vi "_File Server.vi"(4 "Sample Info":string[](array[string]), 5 "AcqMethod":T1[](array[typedef]) {"ScanType" format="%#.6g"; "Mass Range"."Res" items=["High/High", "Medium/Medium", "Low/Low", "High/Medium", "High/Low", "Medium/High", "Medium/Low", "Low/High", "Low/Medium"]}, 7 "file path":path, 8 "error in (no error)":errorcluster, 9 "Scan#":i32=1, 10 "Spectrum":u32[](array[numeric]), 11 "File Command":T6) -> (0 "error out":errorcluster, 1 "Spectrum Out":u32[](array[numeric]), 2 "TIC":u32, 3 "AcqMethod 2":T1[](array[typedef]) {"ScanType" format="%#.6g"; "Mass Range"."Res" items=["High/High", "Medium/Medium", "Low/Low", "High/Medium", "High/Low", "Medium/High", "Medium/Low", "Low/High", "Low/Medium"]}, 6 "Scan# out":i32=1)   [LabVIEW 2015]
doc: "This vi maintains a datalog file for plate positions in motor steps.\nEach datalog record consists of the following data members:\nData/time in secs from 12am 1/1/1904.\nHorizontal motor steps\nVertical motor steps\nAll numbers are stored as 8-byte doubles."
uses:
  Type/_File Command.ctl
  Type/_XML Expt.ctl
  Type/_XML Lens.ctl
  Type/_Mass Range Property.ctl
  Type/_Mass Range Parameters.ctl
  Type/_RT Res Type.ctl
  Configuration/_Global Configuration.vi
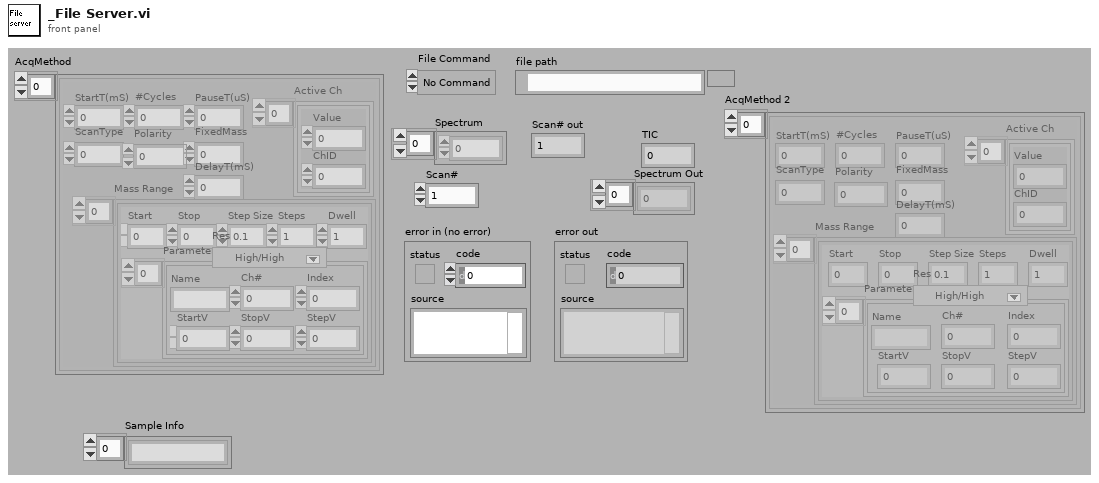
[diagram p1: front panel]
types:
  T1 = typedef "_XML Expt.ctl" = cluster{"StartT(mS)":i32, "#Cycles":i32, "PauseT(uS)":i32, "ScanType":i32, "Polarity":u8, "FixedMass":dbl, "DelayT(mS)":i32, "Active Ch":T2[], "Mass Range":T3[]}
  T2 = typedef "_XML Lens.ctl" = cluster{"Value":dbl, "ChID":u8}
  T3 = typedef "_Mass Range Property.ctl" = cluster{"Start":dbl, "Stop":dbl, "Step Size":dbl, "Steps":i32, "Dwell":dbl, "Parameters":T4[], "Res":T5}
  T4 = typedef "_Mass Range Parameters.ctl" = cluster{"Name":string, "Ch#":u8, "StartV":dbl, "StopV":dbl, "StepV":dbl, "Index":u8}
  T5 = typedef "_RT Res Type.ctl" = u16
  T6 = typedef "_File Command.ctl" = enum16{"No Command", "Open", "Open Read", "Write", "Get Spectrum", "Close"}
  T7 = enum16{"open", "replace", "create", "open or create", "replace or create", "replace or create with confirmation"}
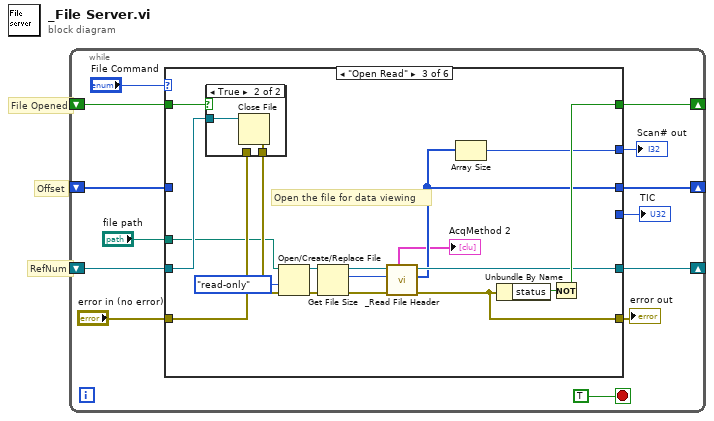
[diagram p0: block diagram]
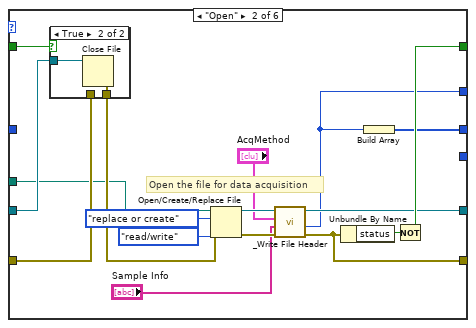
[diagram p3: hidden frame]
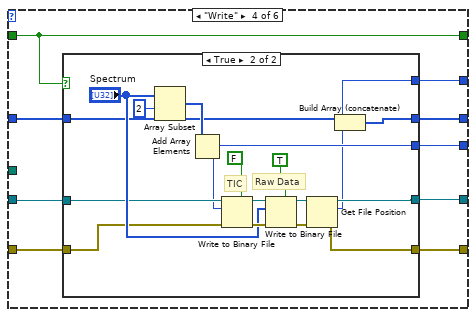
[diagram p6: hidden frame]
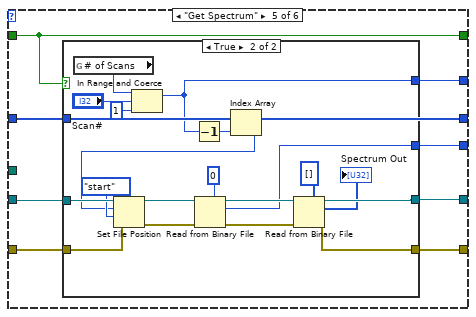
[diagram p8: hidden frame]
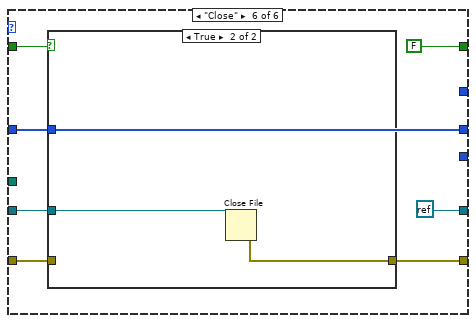
[diagram p10: hidden frame]
diagram:
  # "Offset"
  # "File Opened"
  # "RefNum"
  n1 = while {
    shift-left: _ -> [w8]
    shift-right: [w9] -> _
    shift-left: _ -> [w10]
    shift-right: [w11] -> _
    shift-right: [w5] -> _
    shift-left: _ -> [w4]
    stop <- TRUE stop-if-true
    n2 = case shown="\"Open Read\"" "File Command" {
      tunnel: [w17 w27 w48 w66 w94 refnum<k0> refnum] -> w11
      tunnel: w10 -> [w17 w31 w52 w67 w95 w122]
      tunnel: [w16 w33 w54 w65 w93 FALSE ("Record")] -> w9
      tunnel: w8 -> [w16 w32 w53 w65 w93 w123]
      tunnel: "error in (no error)" -> [w15 w30 w51 w64 w92 w121]
      tunnel: [w15 w26 w45 w63 w91 w120] -> w6
      tunnel: [w14 w21 w40 w61 w90 w119] -> w5
      tunnel: w4 -> [w14 _ _ w62 w90 w119]
      tunnel: "file path" -> [_ w28 w49 _ _ _]
      tunnel: [_ w20 w39 w59 w89 _] -> w2
      tunnel: [_ _ _ w60 w88 _] -> w1
      frame "No Command", Default {
      }
      frame "Open" {
        # "Open the file for data acquisition"
        n3 = case shown="True" w32 {
          tunnel: w31 -> [_ w37]
          tunnel: [w35 w36] -> w29
          tunnel: w30 -> [w35 _]
          frame False {
          }
          frame True {
            n4 = Close File(refnum=w37) -> (error out=w36:errorcluster)  [unwired: 1 in, 1 out]
          }
        }
        n5 = Open/Create/Replace File(file path (use dialog)=w28, error in=w29, operation (0:open)=T7."replace or create", access (0:read/write)=enum16{"read/write", "read-only", "write-only"}."read/write") -> (refnum out=w25:refnum<file>, error out=w24:errorcluster)  [unwired: 3 out]
        n6 = call "_Write File Header.vi"("error in (no error)"=w24, "Sample Info"="Sample Info", "AcqMethod"="AcqMethod", "File Refnum In"=w25) -> ("error out"=w26:errorcluster, "offset"=w20:i64, "File Refnum Out"=w27:refnum<file>)  [unwired: 1 out]
        n7 = Unbundle By Name(w26) -> ("status"=w34:bool)
        n8 = Build Array(w20) -> (w21:i64[])
        n9 = Not(x=w34) -> (.not. x?=w33:bool)
      }
      frame "Open Read" {
        # "Open the file for data viewing"
        n10 = case shown="True" w53 {
          tunnel: w52 -> [_ w58]
          tunnel: [w56 w57] -> w50
          tunnel: w51 -> [w56 _]
          frame False {
          }
          frame True {
            n11 = Close File(refnum=w58) -> (error out=w57:errorcluster)  [unwired: 1 in, 1 out]
          }
        }
        n12 = Open/Create/Replace File(file path (use dialog)=w49, error in=w50, access (0:read/write)=enum16{"read/write", "read-only", "write-only"}."read-only") -> (refnum out=w44:refnum<file>, error out=w43:errorcluster)  [unwired: 4 out]
        n13 = Get File Size ("EOF")(file=w44, error in=w43) -> (refnum out=w47:refnum<file>, size (in bytes)=w41:i64, 0:w46:errorcluster)
        n14 = call "_Read File Header.vi"("error in (no error)"=w46, "File Size"=w41, "File Refnum In"=w47) -> ("error out"=w45:errorcluster, "Offsets"=w40:i64[], "File Refnum Out"=w48:refnum<file>, "AcqMethod"=→"AcqMethod 2":T1[])  [unwired: 2 out]
        n15 = Array Size(array=w40) -> (size(s)=w39:i32)
        n16 = Unbundle By Name(w45) -> ("status"=w55:bool)
        n17 = Not(x=w55) -> (.not. x?=w54:bool)
      }
      frame "Write" {
        n18 = case shown="True" w65 {
          tunnel: w67 -> [w70 w77]
          tunnel: [w70 w85] -> w66
          tunnel: w64 -> [w69 w74]
          tunnel: [w69 w84] -> w63
          tunnel: w62 -> [w68 w75]
          tunnel: [w68 w73] -> w61
          tunnel: [_ w72] -> w60
          tunnel: [_ w71] -> w59
          frame False {
          }
          frame True {
            # "Raw Data"
            # "TIC"
            n19 = Array Subset(array="Spectrum", index=2) -> (w78:u32[])  [unwired: 1 in]
            n20 = Add Array Elements(numeric array=w78) -> (sum=w72:u32)
            n21 = Write to Binary File(file (use dialog)=w77, data=w72, error in=w74, 5:FALSE ("prepend array or string size? (T)")) -> (refnum out=w87:refnum<file>, error out=w86:errorcluster)  [unwired: 3 out]
            n22 = Write to Binary File(file (use dialog)=w87, data="Spectrum", error in=w86, 5:TRUE ("prepend array or string size? (T)")) -> (refnum out=w83:refnum<file>, error out=w82:errorcluster)  [unwired: 3 out]
            n23 = Get File Position(4:w82, 7:w83) -> (0:w84:errorcluster, 2:w71:i64, 3:w85:refnum<file>)
            n24 = Build Array (concatenate)(w75, w71) -> (w73:i64[])
          }
        }
      }
      frame "Get Spectrum" {
        n25 = case shown="True" w93 {
          tunnel: w95 -> [w97 w117]
          tunnel: [w97 w112] -> w94
          tunnel: w92 -> [w96 w116]
          tunnel: [w96 w111] -> w91
          tunnel: w90 -> [_ w104]
          tunnel: [_ w99] -> w89
          tunnel: [_ w98] -> w88
          frame False {
          }
          frame True {
            n26 = global read "_Global Configuration.vi" "# of Scans"() -> (w107:i32)
            n27 = In Range and Coerce(upper limit=w107, x="Scan#", lower limit=1) -> (coerced(x)=w99:i32)  [unwired: 1 out]
            n28 = Decrement(x=w99) -> (x-1=w102:i32)
            n29 = Index Array(array=w104, index=w102) -> (element=w103:i64)
            n30 = Set File Position(offset (in bytes) (0)=w103, refnum=w117, from (0:start)=enum16{"start", "end", "current"}."start" ("pos mode (0:2)"), error in=w116) -> (refnum out=w106:refnum<file>, error out=w105:errorcluster)
            n31 = Read from Binary File(5:u32 0, 8:w105, 11:w106) -> (0:w113:errorcluster, 2:w98:u32, 3:w114:refnum<file>)  [unwired: 4 out]
            n32 = Read from Binary File(5:u32[] [] ("Spectrum"), 8:w113, 11:w114) -> (0:w111:errorcluster, 2:→"Spectrum Out":u32[], 3:w112:refnum<file>)  [unwired: 4 out]
          }
        }
      }
      frame "Close" {
        n33 = case shown="True" w123 {
          tunnel: w122 -> [_ w126]
          tunnel: w121 -> [w125 _]
          tunnel: [w125 w127] -> w120
          tunnel: w119 -> [_ _]
          frame False {
          }
          frame True {
            n34 = Close File(refnum=w126) -> (error out=w127:errorcluster)  [unwired: 1 in, 1 out]
          }
        }
      }
    }
    "error out" <- w6
    "Scan# out" <- w2
    "TIC" <- w1
  }
